vi "Wyznaczenie odległości robota od bazy na podstawie współrzędnych inne roboty.vi"(7 "Azymut robota\n pocz/nowy":dbl caption="Azymut robota pocz/nowy" min=0.0 max=360.0, 9 "Lokalizacja robota GPS":cluster{"Longitude":dbl, "latitude":dbl}, 10 "Parametry odwzorowania Ziemi (WGS84)":cluster{"a":dbl, "b":dbl}={"a"=6378137.0, "b"=6356752.3142} {"b" format="%#.6g"; "a" format="%#.6g"}, 11 "Pocz. poł.":T1 {"UTM"."N [m]" format="%#_10g"}) -> (2 "Rzeczywista odległość robota od startu [m]":cluster{"X [m]":dbl, "Y [m]":dbl}, 3 "Aktualne położenie":T2 {"Szerokośc geograficzna - GPS" format="%_9f"; "Długość geograficzna - GPS" format="%_9f"; "Położenie \nrobota  UTM"."E [m]" format="%#_10g"; "Położenie \nrobota  UTM"."N [m]" format="%#_12g"})   [LabVIEW 2015, in "Biblioteka moduł map v3.lvlib" / "Pomocnicze.lvlib"]
doc: "Zadaniem pliku jest wyznaczenie odległości robota od punktu startowego na podstawie znanych współrzędnych geograficznych pliku startowego oraz odczytów z odbiornika GPS."
uses:
  Pomocnicze.lvlib
  Matematyczne/Matematyczne.lvlib
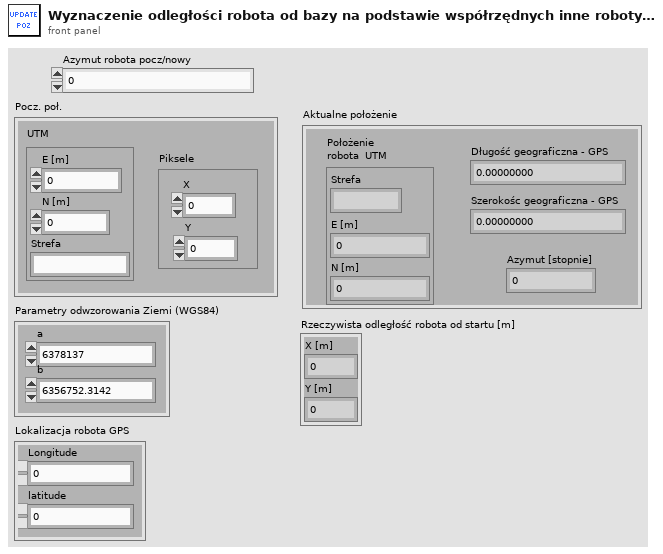
[diagram p1: front panel]
types:
  T1 = cluster{"UTM":cluster{"E [m]":dbl, "N [m]":dbl, "Strefa":string}, "Piksele":cluster{"X":i32, "Y":i32}}
  T2 = cluster{"Położenie \nrobota  UTM":cluster{"E [m]":ext, "N [m]":ext, "Strefa":string}, "Długość geograficzna - GPS":dbl, "Szerokośc geograficzna - GPS":dbl, "Azymut [stopnie]":dbl}
  T3 = cluster{"E [m]":ext, "N [m]":ext, "Strefa":string}
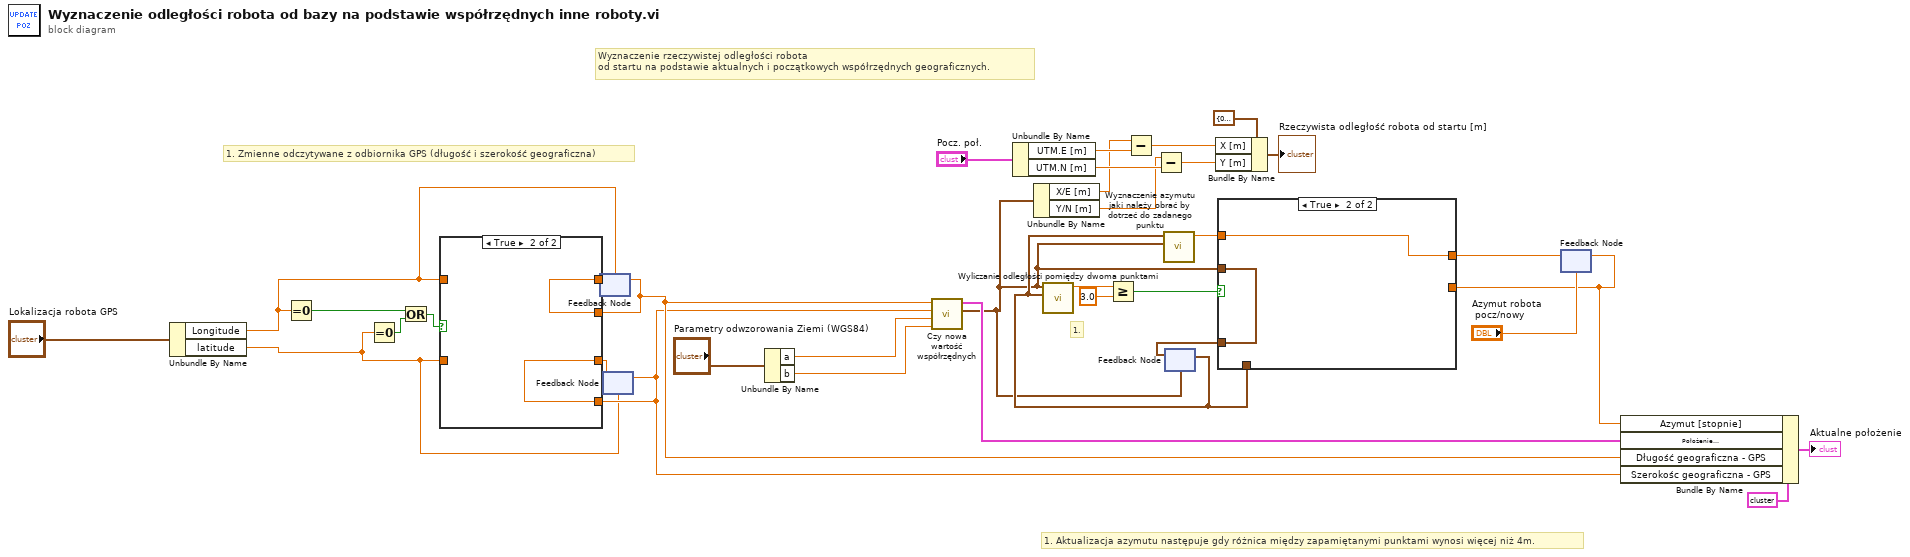
[diagram p0: block diagram]
diagram:
  # "1. Aktualizacja azymutu następuje gdy różnica między zapamiętanymi punktami wynosi więcej niż 4m."
  # "1."
  # "Wyznaczenie rzeczywistej odległości robota \nod startu na podstawie aktualnych i początkowych współrzędnych geograficznych."
  # "1. Zmienne odczytywane z odbiornika GPS (długość i szerokość geograficzna)"
  n1 = Unbundle By Name("Lokalizacja robota GPS") -> ("Longitude"=w2:dbl, "latitude"=w1:dbl)
  n2 = Equal To 0?(x=w2) -> (x = 0?=w11:bool)
  n3 = Equal To 0?(x=w1) -> (x = 0?=w10:bool)
  n4 = Or(x=w11, y=w10) -> (x .or. y?=w9:bool)
  n5 = feedback #1(w2) -> (w6:dbl)
  n6 = feedback #2(w1) -> (w5:dbl)
  n7 = case shown="True" w9 {
    tunnel: [w37 w39] -> w8
    tunnel: w2 -> [w37 _]
    tunnel: w1 -> [w36 _]
    tunnel: [w36 w38] -> w7
    tunnel: w6 -> [_ w39]
    tunnel: w5 -> [_ w38]
    frame False {
    }
    frame True {
    }
  }
  n8 = feedback-in #1(w8) -> ()
  n9 = feedback-in #2(w7) -> ()
  n10 = Unbundle By Name("Parametry odwzorowania Ziemi (WGS84)") -> ("a"=w33:dbl, "b"=w34:dbl)
  n11 = call "Czy nowa wartość współrzędnych.vi"("b"=w34, "a"=w33, "szerokość geograficzna"=w5, "Długość geograficzna"=w6) -> ("Położenie"=w13:cluster{"X/E [m]":dbl, "Y/N [m]":dbl}, "Położenie \nrobota  UTM"=w30:T3)  [unwired: 5 in, 1 out]
  n12 = Unbundle By Name("Pocz. poł.") -> ("UTM.E [m]"=w28:dbl, "UTM.N [m]"=w27:dbl)
  n13 = Unbundle By Name(w13) -> ("X/E [m]"=w26:dbl, "Y/N [m]"=w25:dbl)
  n14 = Subtract(x=w26, y=w28) -> (x-y=w16:dbl)
  n15 = Subtract(x=w25, y=w27) -> (x-y=w15:dbl)
  n16 = feedback #3(w13) -> (w14:cluster{"X/E [m]":dbl, "Y/N [m]":dbl})
  n17 = call "Wyliczanie odległości pomiędzy dwoma punktami.vi"("Polozenie 1"=w14, "Polozenie in"=w13) -> ("Numeric"=w24:dbl)  [unwired: 9 in]
  n18 = Greater Or Equal?(x=w24, y=3.0) -> (x >= y?=w22:bool)
  n19 = call "Wyznaczenie azymutu jaki należy obrać by dotrzeć do zadanego punktu.vi"("Położenie końcowe"=w13, "Położenie aktualne"=w14) -> ("Azymut"=w21:dbl)  [unwired: 9 in]
  n20 = Bundle By Name(cluster=cluster{"X [m]":dbl, "Y [m]":dbl} {"X [m]"=0.0, "Y [m]"=0.0} ("event data"), "X [m]"=w16, "Y [m]"=w15) -> (→"Rzeczywista odległość robota od startu [m]":cluster{"X [m]":dbl, "Y [m]":dbl})
  n21 = feedback #4("Azymut robota\n pocz/nowy") -> (w4:dbl)
  n22 = case shown="True" w22 {
    tunnel: [w40 w43] -> w20
    tunnel: w21 -> [_ w43]
    tunnel: [w41 w42] -> w19
    tunnel: w13 -> [_ w42]
    tunnel: w14 -> [w41 _]
    tunnel: w4 -> [w40 _]
    frame False {
    }
    frame True {
    }
  }
  n23 = feedback-in #3(w19) -> ()
  n24 = feedback-in #4(w20) -> ()
  n25 = Bundle By Name(cluster=T2 {"Położenie \nrobota  UTM"={"E [m]"=0.0, "N [m]"=0.0, "Strefa"=""}, "Długość geograficzna - GPS"=0.0, "Szerokośc geograficzna - GPS"=0.0, "Azymut [stopnie]"=0.0} ("Aktualne położenie"), "Azymut [stopnie]"=w4, "Położenie \nrobota  UTM"=w30, "Długość geograficzna - GPS"=w6, "Szerokośc geograficzna - GPS"=w5) -> (→"Aktualne położenie":T2)
